vi "CAN_SDO.vi"() -> ()   [LabVIEW 2020]
uses:
  <vilib>/CANopenLib/CANOPEN.llb/CANopen Interface Create.vi
  <vilib>/CANopenLib/CANOPEN.llb/CANopen SDO Create.vi
  <vilib>/CANopenLib/CANOPEN.llb/CANopen SDO Write [U16].vi
  <vilib>/CANopenLib/CANOPEN.llb/CANopen SDO Close.vi
  <vilib>/CANopenLib/CANOPEN.llb/CANopen Interface Close.vi
panel:
  out "description":string
  out "completion code":u32 format="%.0x"
  in  "write data":u32=1
  in  "sub-index":u8 format="%.0x"
  in  "object index":u16=24576 format="%.0x"
  in  "node-ID":u8=1 min=1 max=127 step=1
  in  "baud rate":u32(ring)=2 items=["1 Mbit/s"=0, "800 kbit/s"=1, "500 kbit/s"=2, "250 kbit/s"=3, "125 kbit/s"=4, "50 kbit/s"=6, "20 kbit/s"=7, "10 kbit/s"=8]
  in  "CANopen interface":u32(ring)=2 items=["CANopen01", "CANopen02", "CANopen03", "CANopen04", "CANopen05", "CANopen06", "CANopen07", "CANopen08", "CANopen09", "CANopen10", "CANopen11", "CANopen12", "CANopen13", "CANopen14", "CANopen15", "CANopen16", "CANopen17", "CANopen18", "CANopen19", "CANopen20", "CANopen21", "CANopen22", "CANopen23", "CANopen24", "CANopen25", "CANopen26", "CANopen27", "CANopen28", "CANopen29", "CANopen30", "CANopen31", "CANopen32"]
  # "CAN通信倒序"
  # "修改方向为逆时针\nCANID:601\nDATA: 2B 00 60 00 （01） 00 00 00\n\n\nwrite data项类型为u16\n最后需要关闭节点"
  # "修改ID为 2\nCANID:601\nDATA: 2F 01 30 00 （02） 00 00 00\nwrite data项类型为u8\n最后需要复位节点"
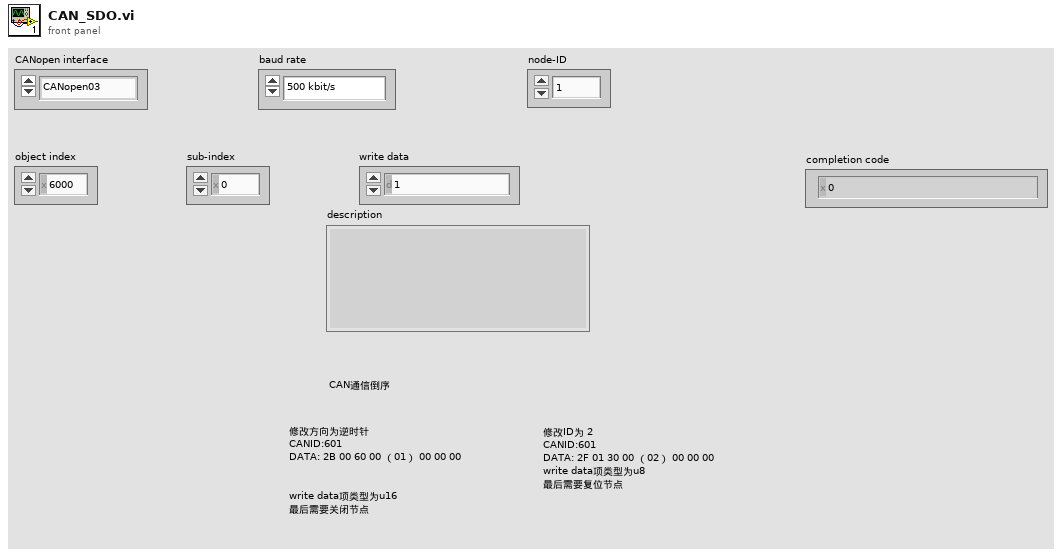
[diagram p1: front panel]
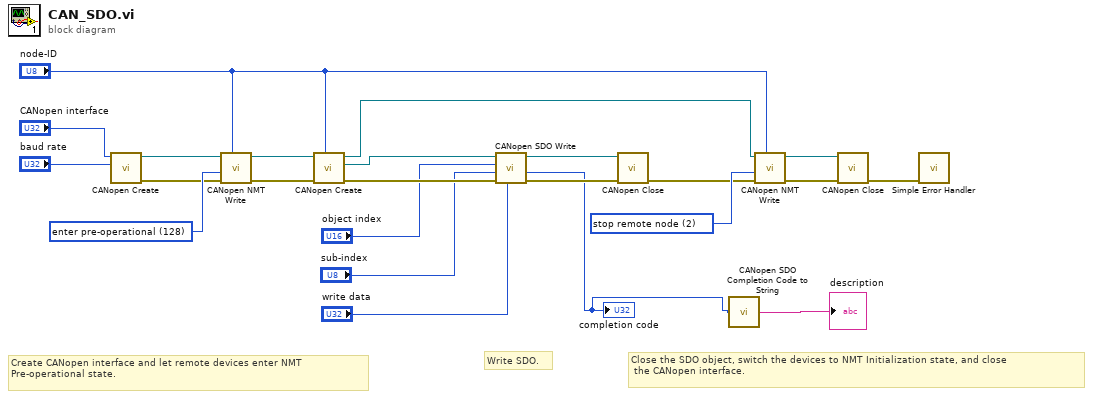
[diagram p0: block diagram]
diagram:
  w13 = u16 2 items=["start remote node"=1, "stop remote node"=2, "enter pre-operational"=128, "reset node"=129, "reset communication"=130] ("command")
  w19 = u16 128 items=["start remote node"=1, "stop remote node"=2, "enter pre-operational"=128, "reset node"=129, "reset communication"=130] ("command")
  # "Create CANopen interface and let remote devices enter NMT\nPre-operational state."
  # "Write SDO."
  # "Close the SDO object, switch the devices to NMT Initialization state, and close\n the CANopen interface."
  n1 = call-poly <vilib>:"CANopen Create.vi"("baud rate"="baud rate", "interface name"="CANopen interface") -> ("error out"=w5:errorcluster, "interface object out"=w18:refnum<k20>)  [unwired: 8 in]
  n2 = call <vilib>:"CANopen NMT Write.vi"("node-ID (0)"="node-ID", "error in (no error)"=w5, "command"=w19, "interface object in"=w18) -> ("error out"=w22:errorcluster, "interface object out"=w23:refnum<k20>)  [unwired: 6 in]
  n3 = call-poly <vilib>:"CANopen Create.vi"("node-ID"="node-ID", "error in (no error)"=w22, "interface object in"=w23) -> ("error out"=w17:errorcluster, "SDO object out"=w4:refnum<k20>, "interface object out"=w14:refnum<k20>)  [unwired: 6 in]
  n4 = call-poly <vilib>:"CANopen SDO Write.vi"("U16 data"="write data", "error in (no error)"=w17, "object sub-index (0)"="sub-index", "object index"="object index", "SDO object in"=w4) -> ("error out"=w11:errorcluster, "completion code"=w2:u32, "SDO object out"=w9:refnum<k20>)  [unwired: 4 in]
  "completion code" <- w2
  n5 = call-poly <vilib>:"CANopen Close.vi"("error in (no error)"=w11, "SDO object in"=w9) -> ("error out"=w10:errorcluster)  [unwired: 9 in]
  n6 = call <vilib>:"CANopen SDO Completion Code to String.vi"("SDO completion code"=w2) -> ("description"=→"description":string)
  n7 = call <vilib>:"CANopen NMT Write.vi"("node-ID (0)"="node-ID", "error in (no error)"=w10, "command"=w13, "interface object in"=w14) -> ("error out"=w8:errorcluster, "interface object out"=w7:refnum<k20>)  [unwired: 6 in]
  n8 = call-poly <vilib>:"CANopen Close.vi"("error in (no error)"=w8, "interface object in"=w7) -> ("error out"=w6:errorcluster)  [unwired: 9 in]
  n9 = call <vilib>:"Simple Error Handler.vi"("error in (no error)"=w6) -> ()  [unwired: 4 in, 5 out]
